vi "time_of_last_0.vi"(8 "time":dbl format="%#_13g", 9 "t_start":dbl format="%#_13g", 11 "Frequency (Hz)":dbl format="%#_13g") -> (1 "Number of zeroes":i32, 2 "time since last 0":dbl)   [LabVIEW 2016]
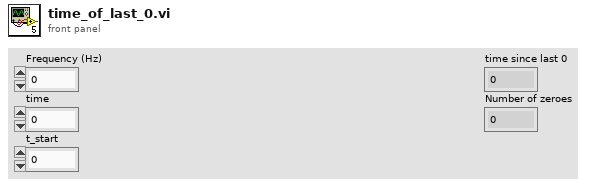
[diagram p1: front panel]
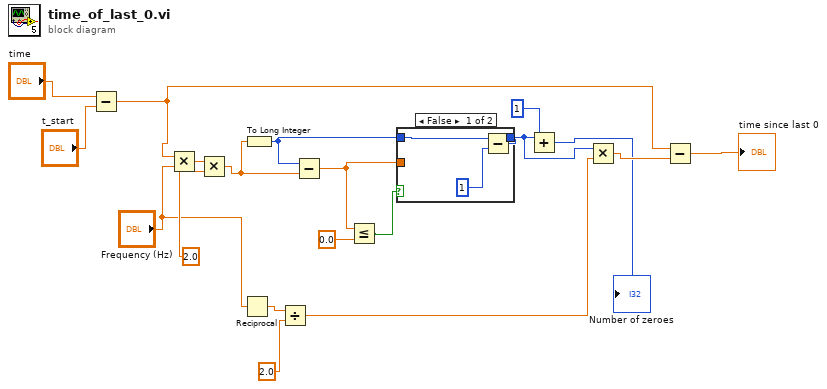
[diagram p0: block diagram]
diagram:
  n1 = Subtract(x="time", y="t_start") -> (x-y=w7:dbl)
  n2 = Multiply(x=w7, y="Frequency (Hz)") -> (x*y=w16:dbl)
  n3 = Multiply(x=w16, y=2.0) -> (x*y=w14:dbl)
  n4 = Reciprocal(x="Frequency (Hz)") -> (1/x=w12:dbl)
  n5 = To Long Integer(number=w14) -> (32bit integer=w19:i32)
  n6 = Divide(x=w12, y=2.0) -> (x/y=w10:dbl)
  n7 = Subtract(x=w19, y=w14) -> (x-y=w4:dbl)
  n8 = Less Or Equal?(x=w4, y=0.0) -> (x <= y?=w5:bool)
  n9 = case shown="False" w5 {
    tunnel: w4 -> [_ _]
    tunnel: w19 -> [w22 w23]
    tunnel: [w20 w23] -> w2
    frame False {
      n10 = Subtract(x=w22, y=1) -> (x-y=w20:i32)
    }
    frame True {
    }
  }
  n11 = Add(x=w2, y=1) -> (x+y=→"Number of zeroes":i32)
  n12 = Multiply(x=w2, y=w10) -> (x*y=w18:dbl)
  n13 = Subtract(x=w7, y=w18) -> (x-y=→"time since last 0":dbl)
